vi "plotINIT.vi"(5 "Plot Buffer Size":u32=10) -> (0 "Pin":bool[](array[boolean]), 1 "Data Array output":dbl[][](array[numeric]) format="%.2f", 2 "X-Axis Array output":dbl[][](array[numeric]) format="%.2f", 3 "File Info Buffer Out":T1[](array[typedef])=[{"FilePath"=path "", "Field (T)"=0.0, "Temperature (K)"=0.0, "X-Axis"=enum."Point", "Center nm"=0.0, "Current Grating Density"=enum."150", "CCD Parameters"={"Exposure Time (s)"=0.2, "Offset"=0.0, "BkgrdCrct"=FALSE, "Shutter"=FALSE, "Mode"=enum."Regular", "Repetition"=4, "dt or s"=0.0}, "Operation Mode"=enum."Standby", "Exp Index"=0, "Index_repetition"=0, "Index"=0, "Current Detector"=enum."CCD-1024x256"}, {"FilePath"=path "", "Field (T)"=0.0, "Temperature (K)"=0.0, "X-Axis"=enum."Point", "Center nm"=0.0, "Current Grating Density"=enum."150", "CCD Parameters"={"Exposure Time (s)"=0.2, "Offset"=0.0, "BkgrdCrct"=FALSE, "Shutter"=FALSE, "Mode"=enum."Regular", "Repetition"=4, "dt or s"=0.0}, "Operation Mode"=enum."Standby", "Exp Index"=0, "Index_repetition"=0, "Index"=0, "Current Detector"=enum."CCD-1024x256"}, {"FilePath"=path "", "Field (T)"=0.0, "Temperature (K)"=0.0, "X-Axis"=enum."Point", "Center nm"=0.0, "Current Grating Density"=enum."150", "CCD Parameters"={"Exposure Time (s)"=0.2, "Offset"=0.0, "BkgrdCrct"=FALSE, "Shutter"=FALSE, "Mode"=enum."Regular", "Repetition"=4, "dt or s"=0.0}, "Operation Mode"=enum."Standby", "Exp Index"=0, "Index_repetition"=0, "Index"=0, "Current Detector"=enum."CCD-1024x256"}, {"FilePath"=path "", "Field (T)"=0.0, "Temperature (K)"=0.0, "X-Axis"=enum."Point", "Center nm"=0.0, "Current Grating Density"=enum."150", "CCD Parameters"={"Exposure Time (s)"=0.2, "Offset"=0.0, "BkgrdCrct"=FALSE, "Shutter"=FALSE, "Mode"=enum."Regular", "Repetition"=4, "dt or s"=0.0}, "Operation Mode"=enum."Standby", "Exp Index"=0, "Index_repetition"=0, "Index"=0, "Current Detector"=enum."CCD-1024x256"}, {"FilePath"=path "", "Field (T)"=0.0, "Temperature (K)"=0.0, "X-Axis"=enum."Point", "Center nm"=0.0, "Current Grating Density"=enum."150", "CCD Parameters"={"Exposure Time (s)"=0.2, "Offset"=0.0, "BkgrdCrct"=FALSE, "Shutter"=FALSE, "Mode"=enum."Regular", "Repetition"=4, "dt or s"=0.0}, "Operation Mode"=enum."Standby", "Exp Index"=0, "Index_repetition"=0, "Index"=0, "Current Detector"=enum."CCD-1024x256"}, {"FilePath"=path "", "Field (T)"=0.0, "Temperature (K)"=0.0, "X-Axis"=enum."Point", "Center nm"=0.0, "Current Grating Density"=enum."150", "CCD Parameters"={"Exposure Time (s)"=0.2, "Offset"=0.0, "BkgrdCrct"=FALSE, "Shutter"=FALSE, "Mode"=enum."Regular", "Repetition"=4, "dt or s"=0.0}, "Operation Mode"=enum."Standby", "Exp Index"=0, "Index_repetition"=0, "Index"=0, "Current Detector"=enum."CCD-1024x256"}, {"FilePath"=path "", "Field (T)"=0.0, "Temperature (K)"=0.0, "X-Axis"=enum."Point", "Center nm"=0.0, "Current Grating Density"=enum."150", "CCD Parameters"={"Exposure Time (s)"=0.2, "Offset"=0.0, "BkgrdCrct"=FALSE, "Shutter"=FALSE, "Mode"=enum."Regular", "Repetition"=4, "dt or s"=0.0}, "Operation Mode"=enum."Standby", "Exp Index"=0, "Index_repetition"=0, "Index"=0, "Current Detector"=enum."CCD-1024x256"}, {"FilePath"=path "", "Field (T)"=0.0, "Temperature (K)"=0.0, "X-Axis"=enum."Point", "Center nm"=0.0, "Current Grating Density"=enum."150", "CCD Parameters"={"Exposure Time (s)"=0.2, "Offset"=0.0, "BkgrdCrct"=FALSE, "Shutter"=FALSE, "Mode"=enum."Regular", "Repetition"=4, "dt or s"=0.0}, "Operation Mode"=enum."Standby", "Exp Index"=0, "Index_repetition"=0, "Index"=0, "Current Detector"=enum."CCD-1024x256"}, {"FilePath"=path "/Opticsmac/Documents/Data", "Field (T)"=999.0, "Temperature (K)"=300.0, "X-Axis"=enum."Point", "Center nm"=600.0, "Current Grating Density"=enum."150", "CCD Parameters"={"Exposure Time (s)"=0.2, "Offset"=0.0, "BkgrdCrct"=FALSE, "Shutter"=FALSE, "Mode"=enum."Regular", "Repetition"=4, "dt or s"=0.0}, "Operation Mode"=enum."NML Data Acquisition", "Exp Index"=0, "Index_repetition"=0, "Index"=0, "Current Detector"=enum."CCD-1024x256"}, {"FilePath"=path "", "Field (T)"=0.0, "Temperature (K)"=0.0, "X-Axis"=enum."Point", "Center nm"=0.0, "Current Grating Density"=enum."150", "CCD Parameters"={"Exposure Time (s)"=0.2, "Offset"=0.0, "BkgrdCrct"=FALSE, "Shutter"=FALSE, "Mode"=enum."Regular", "Repetition"=4, "dt or s"=0.0}, "Operation Mode"=enum."Standby", "Exp Index"=0, "Index_repetition"=0, "Index"=0, "Current Detector"=enum."CCD-1024x256"}] {"CCD Parameters"."dt or s" format="%#.6f"; "CCD Parameters"."Repetition" min=1; "CCD Parameters"."Offset" format="%#.2f"; "CCD Parameters"."Exposure Time (s)" min=0.02 max=6000.0 format="%#.2f"; "Center nm" format="%.2f"; "Temperature (K)" format="%.2f"; "Field (T)" format="%.2f"}, 4 "Updated Old Trace?":bool[](array[boolean])=[FALSE, FALSE, FALSE, FALSE, FALSE, FALSE, FALSE, FALSE, FALSE, TRUE])   [LabVIEW 2024]
uses:
  Globals and TypeDefs/Type Definitions.llb/FileInfoParameter.ctt
  Globals and TypeDefs/Type Definitions.llb/Wavelength Unit.ctt
  Globals and TypeDefs/Type Definitions.llb/McPherson Grating Density.ctl
  Globals and TypeDefs/Type Definitions.llb/CCDParameter.ctt
  Globals and TypeDefs/Type Definitions.llb/OperationMode.ctt
  Globals and TypeDefs/Type Definitions.llb/ListOfDetectors.ctt
panel:
  out "X graph":dbl[][](graph)
  out "y graph":dbl[][](graph)
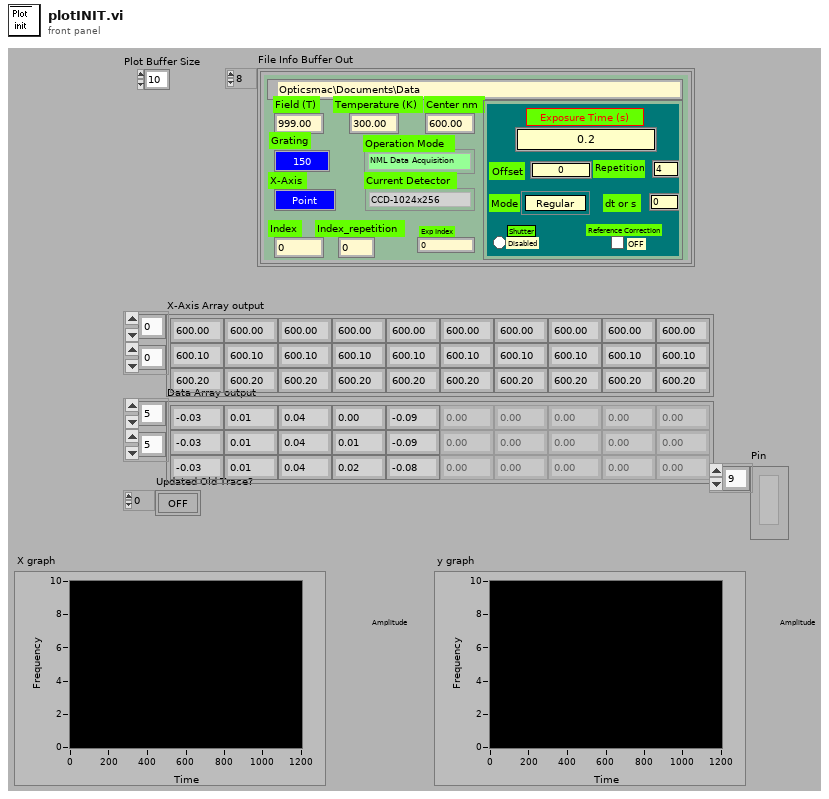
[diagram p1: front panel]
types:
  T1 = typedef "FileInfoParameter.ctt" = cluster{"FilePath":path, "Field (T)":dbl, "Temperature (K)":dbl, "X-Axis":T2, "Center nm":dbl, "Current Grating Density":T3, "CCD Parameters":T4, "Operation Mode":T5, "Exp Index":u32, "Index_repetition":u16, "Index":u16, "Current Detector":T6}
  T2 = typedef "Wavelength Unit.ctt" = enum8{"Point", "nm", "eV", "meV", "cm_1"}
  T3 = typedef "McPherson Grating Density.ctl" = enum8{"150", "300", "600", "1200", "1800"}
  T4 = typedef "CCDParameter.ctt" = cluster{"Exposure Time (s)":dbl, "Offset":dbl, "BkgrdCrct":bool, "Shutter":bool, "Mode":enum8{"Regular", "OverExp Cor", "SpikeRemove", "ForCalibration"}, "Repetition":u16, "dt or s":dbl}
  T5 = typedef "OperationMode.ctt" = enum16{"Standby", "CCD Single Shot", "CCD Sequence Shots", "CCD Custom Shots", "CCD Reference Shot", "Step Scanning ", "Time Scanning", "NML Data Acquisition"}
  T6 = typedef "ListOfDetectors.ctt" = enum8{"CCD-1024x256", "InGaAs PDA-1024x1", "CCD-1340x400", "Ge Single Channel", "Si Single Channel", "PMT Single Channel"}
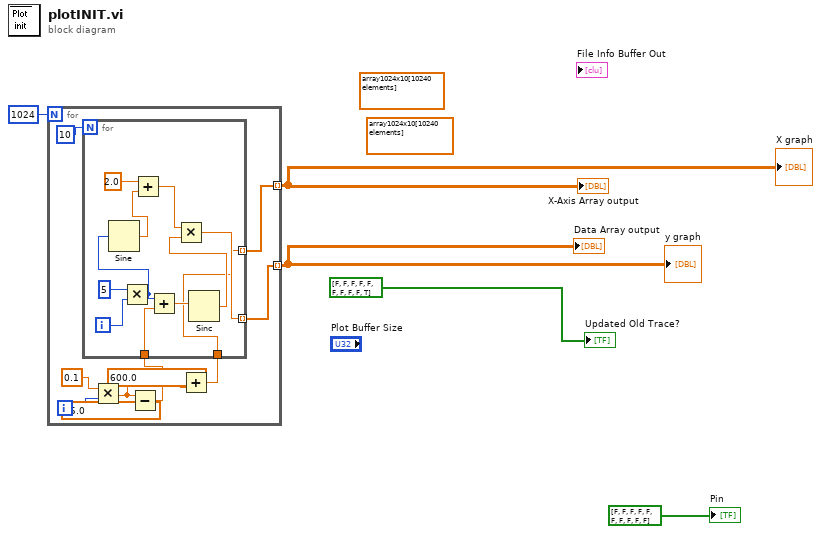
[diagram p0: block diagram]
diagram:
  (unwired) dbl[][] array1024x10[10240 elements] ("X-Axis Array output")
  (unwired) dbl[][] array1024x10[10240 elements] ("Data Array output")
  n1 = for {
    N: 1024 -> [_]
    tunnel: [w14] -> w2 mode=indexing
    tunnel: [w13] -> w3 mode=indexing
    i -> [w11]
    n2 = Multiply(x=0.1, y=w11) -> (x*y=w8:dbl)
    n3 = Subtract(x=w8, y=75.0) -> (x-y=w9:dbl)
    n4 = Add(x=600.0, y=w8) -> (x+y=w6:dbl)
    n5 = for {
      N: 10 -> [_]
      tunnel: [w16] -> w14 mode=indexing
      tunnel: [w17] -> w13 mode=indexing
      tunnel: w9 -> [w24]
      tunnel: w6 -> [w16]
      i -> [w26]
      n6 = Multiply(x=5, y=w26) -> (x*y=w22:i32)
      n7 = Sine(x=w22) -> (sin(x)=w21:dbl)
      n8 = Add(x=2.0, y=w21) -> (x+y=w19:dbl)
      n9 = Add(x=w22, y=w24) -> (x+y=w23:dbl)
      n10 = Sinc(1:w23) -> (0:w18:dbl)
      n11 = Multiply(x=w19, y=w18) -> (x*y=w17:dbl)
    }
  }
  "Data Array output" <- w3
  "X-Axis Array output" <- w2
  "y graph" <- w3
  "X graph" <- w2
  "Updated Old Trace?" <- bool[] [FALSE, FALSE, FALSE, FALSE, FALSE, FALSE, FALSE, FALSE, FALSE, TRUE] ("Updated Old Trace?")
  "Pin" <- bool[] [FALSE, FALSE, FALSE, FALSE, FALSE, FALSE, FALSE, FALSE, FALSE, FALSE] ("Updated Old Trace?")
